vi "To Start and Stop (array).vi"(5 "center/span":T1 {"span" min=0.0 step=10000.0 format="%.2g"; "center" min=0.0 step=10000.0 format="%.2g"}) -> (1 "start/stop":T2 {"stop" min=0.0 step=10000.0 format="%.2g"; "start" min=0.0 step=10000.0 format="%.2g"})   [LabVIEW 2009]
doc: "Takes two bare numbers that indicate the average (\"center\") and difference (\"span\") of two numbers and returns the beginning and end of the range."
uses:
  FG FM sweep start stop control.ctl
  FG FM sweep center span control.ctl
  Math Operations/To Start and Stop (frequency).vi
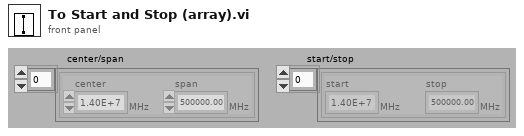
[diagram p1: front panel]
types:
  T1 = typedef "FG FM sweep center span control.ctl" = cluster{"center":dbl[unit], "span":dbl[unit]}[]
  T2 = typedef "FG FM sweep start stop control.ctl" = cluster{"start":dbl[unit], "stop":dbl[unit]}[]
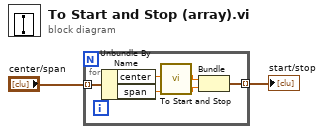
[diagram p0: block diagram]
diagram:
  n1 = for {
    tunnel: "center/span" -> [w8] mode=indexing
    tunnel: [w7] -> w1 mode=indexing
    n2 = Unbundle By Name(w8) -> ("center"=w6:dbl[unit], "span"=w5:dbl[unit])
    n3 = call-poly "To Start and Stop.vi"("span"=w5, "center"=w6) -> ("stop"=w4:dbl[unit], "start"=w3:dbl[unit])  [unwired: 4 out]
    n4 = Bundle("start"=w3, "stop"=w4) -> (w7:cluster{"start":dbl[unit], "stop":dbl[unit]})  [unwired: 1 out]
  }
  "start/stop" <- w1
